vi "Horst-ZeitTest.vi"() -> ()   [LabVIEW 2017]
uses:
  <vilib>/rvi/interface/nirviMethod/nirviMethod.xnode
  E:/HAGAR-V_ECD/FPGA-Programm_ECD.vi
  <vilib>/FPGAPlugInAG/cRIO-9035/niLvFpga_WriteFifo_cRIO-9035.vi
  <vilib>/rvi/errors/niLvFpgaMergeErrorWithErrorCode.vi
  <vilib>/FPGAPlugInAG/cRIO-9035/niLvFpga_ReadFifo_cRIO-9035.vi
  <vilib>/rvi/interface/nirviReadWriteControl/nirviReadWriteControl.xnode
  <vilib>/rvi/interface/nirviCloseFPGA/nirviCloseFPGA.xnode
  <vilib>/regexp/Match Regular Expression.xnode
  GVECDs.vi
  FPGA Bitfiles/HAGAR-VECD_FPGATarget_FPGA-ProgrammECD_J-wKM9Jb3G8.lvbitx
  NiFpgaLv.dll
  <vilib>/Utility/error.llb/Error Cluster From Error Code.vi
  <vilib>/rvi/errors/niLvFpgaAdjustHostInterfaceError.vi
  <vilib>/FPGAPlugInAG/cRIO-9035/niLvFpga_Close_cRIO-9035.vi
panel:
  out "ECD2":string
  out "ECD1":string
  out "Array":errorcluster[](array[cluster])
  out "MW":dbl[](array[numeric])
  out "Fehler":bool[](array[boolean])
  in  "SP":dbl[](array[numeric]) format="%#_13g"
  in  "Stopp":bool
  out "stop":errorcluster caption="Fehler (Ausgang)"
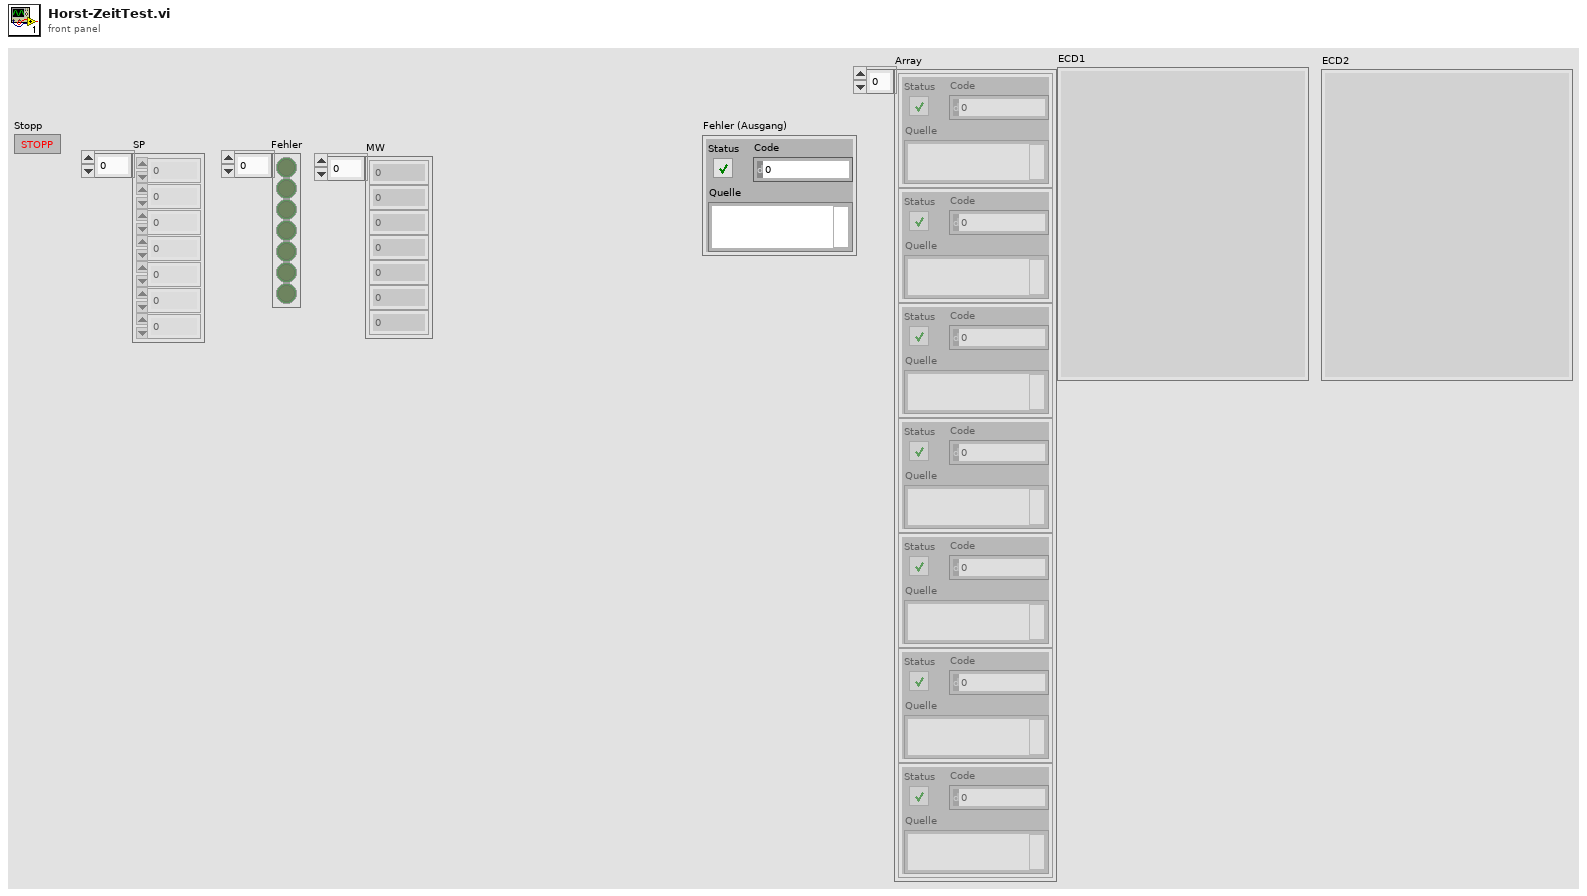
[diagram p1: front panel]
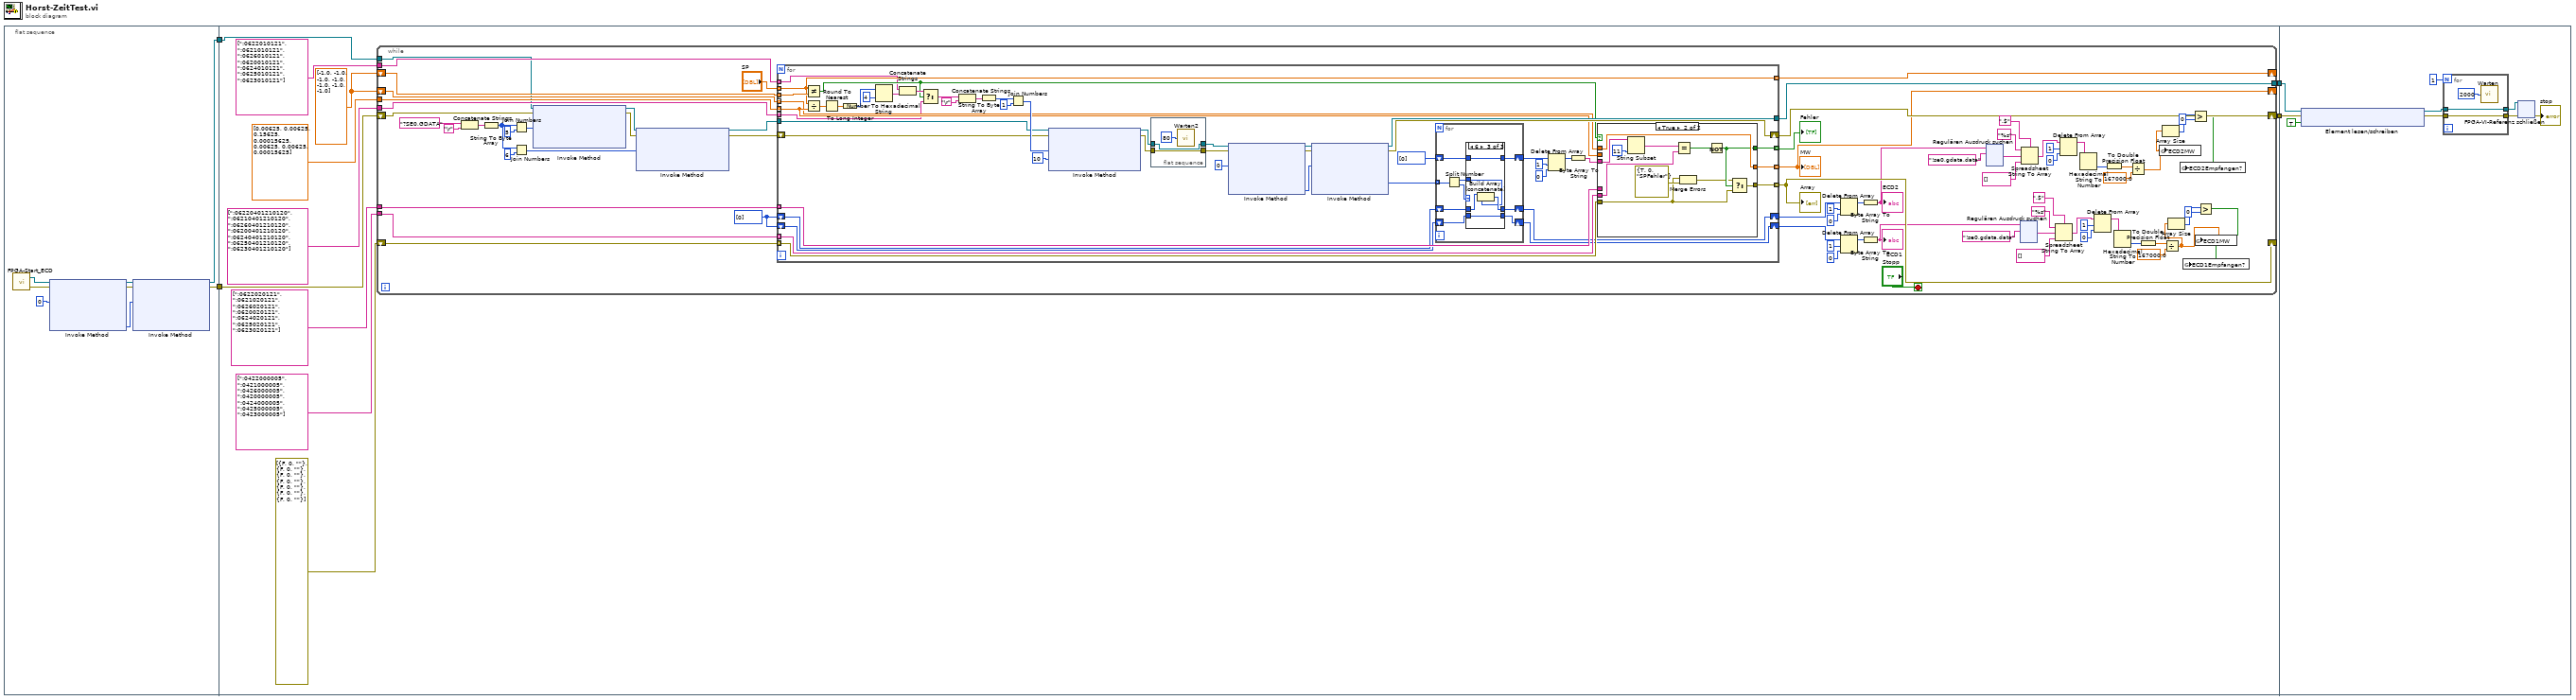
[diagram p0: block diagram]
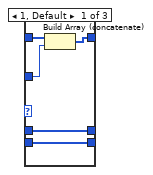
[diagram p2: hidden frame]
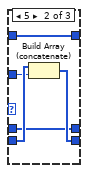
[diagram p3: hidden frame]
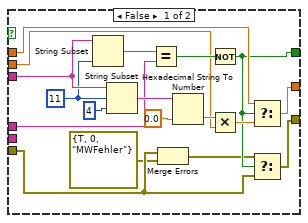
[diagram p4: hidden frame]
diagram:
  n1 = flat-sequence {
    tunnel: [w6] -> w4
    tunnel: [w5] -> w3
    tunnel: [w23] -> w2
    tunnel: [w22] -> w1
    tunnel: w4 -> [w21]
    tunnel: w3 -> [w20]
    tunnel: w2 -> [w425]
    tunnel: w1 -> [w424]
    frame #0 {
      n2 = call "FPGA-Start_ECD.vi"() -> ("error out"=w7:errorcluster, "FPGA-VI-Referenz (Ausgang)"=w8:refnum<k20>)  [unwired: 2 in]
      n3 = xnode "Invoke Method"("FPGA-VI-Referenz (Eingang)"=w8, "Fehler (Eingang)"=w7, "Anzahl der Elemente"=u32 0) -> ("FPGA-VI-Referenz (Ausgang)"=w12:refnum<k20>, "Fehler (Ausgang)"=w9:errorcluster, "Verbleibende Elemente"=w10:u32)  [unwired: 1 in, 1 out]
      n4 = xnode "Invoke Method"("FPGA-VI-Referenz (Eingang)"=w12, "Fehler (Eingang)"=w9, "Anzahl der Elemente"=w10) -> ("FPGA-VI-Referenz (Ausgang)"=w6:refnum<k20>, "Fehler (Ausgang)"=w5:errorcluster)  [unwired: 1 in, 2 out]
    }
    frame #1 {
      w19 = dbl[] [-1.0, -1.0, -1.0, -1.0, -1.0, -1.0, -1.0]
      n5 = while {
        shift-right: [w95] -> w22
        shift-left: w20 -> [w70]
        shift-right: [w92] -> _
        shift-left: w19 -> [w93]
        shift-right: [w89] -> _
        shift-left: w19 -> [w88]
        tunnel: string[] [":0622010121", ":0621010121", ":0626010121", ":0620010121", ":0624010121", ":0625010121", ":0623010121"] ("SPvorgebenMod2A") -> [w87]
        tunnel: string[] [":06220401210120", ":06210401210120", ":06260401210120", ":06200401210120", ":06240401210120", ":06250401210120", ":06230401210120"] ("MWabfragenMod2A") -> [w86]
        tunnel: dbl[] [0.00625, 0.00625, 0.15625, 0.00015625, 0.00625, 0.00625, 0.00015625] ("FaktorMod2A") -> [w85]
        tunnel: string[] [":0622020121", ":0621020121", ":0626020121", ":0620020121", ":0624020121", ":0625020121", ":0623020121"] ("MWAntwortMod2A") -> [w84]
        tunnel: string[] [":0422000005", ":0421000005", ":0426000005", ":0420000005", ":0424000005", ":0425000005", ":0423000005"] ("y") -> [w83]
        shift-right: [w82] -> _
        shift-left: errorcluster[] [{"status"=FALSE, "code"=0, "source"=""}, {"status"=FALSE, "code"=0, "source"=""}, {"status"=FALSE, "code"=0, "source"=""}, {"status"=FALSE, "code"=0, "source"=""}, {"status"=FALSE, "code"=0, "source"=""}, {"status"=FALSE, "code"=0, "source"=""}, {"status"=FALSE, "code"=0, "source"=""}] -> [w81]
        tunnel: w21 -> [w71]
        tunnel: [w96] -> w23
        stop <- "Stopp" stop-if-true
        w80 = u8[] [0]
        n6 = Concatenate Strings("?SE0,GDATA" ("Schreibpuffer"), "\r") -> (w59:string)
        n7 = String To Byte Array(string=w59) -> (unsigned byte array=w58:u8[])
        n8 = Join Numbers(hi=w58, lo=u8 5) -> ((hi.lo)=w63:u16[])
        n9 = Join Numbers(hi=w58, lo=u8 6) -> ((hi.lo)=w62:u16[])
        n10 = xnode "Invoke Method"("FPGA-VI-Referenz (Eingang)"=w71, "Fehler (Eingang)"=w70, "Daten"=w63) -> ("FPGA-VI-Referenz (Ausgang)"=w67:refnum<k20>, "Fehler (Ausgang)"=w65:errorcluster)  [unwired: 1 in, 1 out]
        n11 = xnode "Invoke Method"("FPGA-VI-Referenz (Eingang)"=w67, "Fehler (Eingang)"=w65, "Daten"=w62) -> ("FPGA-VI-Referenz (Ausgang)"=w66:refnum<k20>, "Fehler (Ausgang)"=w64:errorcluster)  [unwired: 1 in, 1 out]
        n12 = for {
          tunnel: w93 -> [w342] mode=indexing
          tunnel: [w338] -> w92 mode=indexing
          tunnel: [w339] -> w91 mode=indexing
          shift-right: [w362] -> w95
          shift-left: w64 -> [w354]
          tunnel: "SP" -> [w338] mode=indexing
          tunnel: w85 -> [w337] mode=indexing
          tunnel: [w336] -> w89 mode=indexing
          tunnel: w88 -> [w335] mode=indexing
          tunnel: w87 -> [w334] mode=indexing
          tunnel: w86 -> [w333] mode=indexing
          tunnel: w84 -> [w332] mode=indexing
          tunnel: w83 -> [w331] mode=indexing
          tunnel: [w330] -> w82 mode=indexing
          tunnel: w81 -> [w329] mode=indexing
          shift-right: [w319] -> w75
          shift-left: w80 -> [w322]
          shift-right: [w320] -> w74
          shift-left: w80 -> [w321]
          tunnel: w66 -> [w355]
          tunnel: [w365] -> w96
          n13 = Not Equal?(x=w338, y=w342) -> (x != y?=w340:bool)
          n14 = Divide(x=w338, y=w337) -> (x/y=w349:dbl)
          n15 = Round To Nearest(number=w349) -> (nearest integer value=w348:dbl)
          n16 = To Long Integer(number=w348) -> (32bit integer=w347:i32)
          n17 = Number To Hexadecimal String(1:i16 4 ("Breite (-)"), 2:w347) -> (0:w345:string)
          n18 = Concatenate Strings(w334, w345) -> (w344:string)
          n19 = Select(t=w344, s=w340, f=w333) -> (s? t:f=w343:string)
          n20 = Concatenate Strings(w343, "\r") -> (w361:string)
          n21 = String To Byte Array(string=w361) -> (unsigned byte array=w359:u8[])
          n22 = Join Numbers(hi=w359, lo=u8 1) -> ((hi.lo)=w360:u16[])
          n23 = xnode "Invoke Method"("FPGA-VI-Referenz (Eingang)"=w355, "Fehler (Eingang)"=w354, "Daten"=w360, "Timeout (ms)"=10) -> ("FPGA-VI-Referenz (Ausgang)"=w353:refnum<k20>, "Fehler (Ausgang)"=w351:errorcluster)  [unwired: 1 out]
          n24 = flat-sequence {
            tunnel: w353 -> [w423]
            tunnel: [w423] -> w352
            tunnel: w351 -> [w422]
            tunnel: [w422] -> w350
            frame #0 {
              n25 = call "Warten2"("Count(mSec)"=u32 80) -> ()  [unwired: 1 out]
            }
          }
          n26 = xnode "Invoke Method"("FPGA-VI-Referenz (Eingang)"=w352, "Fehler (Eingang)"=w350, "Anzahl der Elemente"=u32 0) -> ("FPGA-VI-Referenz (Ausgang)"=w364:refnum<k20>, "Fehler (Ausgang)"=w363:errorcluster, "Verbleibende Elemente"=w366:u32)  [unwired: 1 in, 1 out]
          n27 = xnode "Invoke Method"("FPGA-VI-Referenz (Eingang)"=w364, "Fehler (Eingang)"=w363, "Anzahl der Elemente"=w366) -> ("FPGA-VI-Referenz (Ausgang)"=w365:refnum<k20>, "Fehler (Ausgang)"=w362:errorcluster, "Daten"=w328:u16[])  [unwired: 1 in, 1 out]
          n28 = for {
            tunnel: w328 -> [w376] mode=indexing
            shift-right: [w370] -> w326
            shift-left: u8[] [0] -> [w371]
            shift-right: [w369] -> w319
            shift-left: w322 -> [w372]
            shift-right: [w368] -> w320
            shift-left: w321 -> [w373]
            n29 = Split Number(x=w376) -> (hi(x)=w374:u8, lo(x)=w375:u8)
            n30 = case shown="6" w375 {
              tunnel: w374 -> [w381 w384 w387]
              tunnel: w373 -> [w377 w382 w390]
              tunnel: w372 -> [w378 w385 w389]
              tunnel: w371 -> [w380 w386 w391]
              tunnel: [w379 w386 w391] -> w370
              tunnel: [w378 w383 w389] -> w369
              tunnel: [w377 w382 w388] -> w368
              frame 1, Default {
                n31 = Build Array (concatenate)(w380, w381) -> (w379:u8[])
              }
              frame 5 {
                n32 = Build Array (concatenate)(w385, w384) -> (w383:u8[])
              }
              frame 6 {
                n33 = Build Array (concatenate)(w390, w387) -> (w388:u8[])
              }
            }
          }
          n34 = Delete From Array(array=w326, length=1 ("Länge"), index=0 ("Index")) -> (array with subset deleted=w323:u8[])  [unwired: 1 out]
          n35 = Byte Array To String(unsigned byte array=w323) -> (string=w341:string)
          n36 = case shown="True" w340 {
            tunnel: w341 -> [w407 w420]
            tunnel: [w396 w414] -> w339
            tunnel: w337 -> [w401 _]
            tunnel: [w398 w416] -> w336
            tunnel: w335 -> [w399 w416]
            tunnel: w332 -> [w397 _]
            tunnel: w331 -> [_ w415]
            tunnel: [w395 w413] -> w330
            tunnel: w329 -> [w394 w410]
            frame False {
              w406 = 11 ("Länge (Rest)")
              n37 = String Subset(string=w407, length (rest)=w406) -> (substring=w409:string)  [unwired: 1 in]
              n38 = String Subset(string=w407, offset (0)=w406, length (rest)=4 ("Länge (Rest)")) -> (substring=w404:string)
              n39 = Equal?(x=w409, y=w397) -> (x = y?=w408:bool)
              n40 = Merge Errors(w394, errorcluster {"status"=TRUE, "code"=0, "source"="MWFehler"} ("Fehlerkonstante")) -> (w393:errorcluster)
              n41 = Hexadecimal String To Number(string=w404, default (0uL)=0.0 ("Standard (0 U32)")) -> (number=w402:dbl)  [unwired: 1 in, 1 out]
              n42 = Not(x=w408) -> (.not. x?=w396:bool)
              n43 = Multiply(x=w402, y=w401) -> (x*y=w400:dbl)
              n44 = Select(t=w399, s=w396, f=w400) -> (s? t:f=w398:dbl)
              n45 = Select(t=w393, s=w396, f=w394) -> (s? t:f=w395:errorcluster)
            }
            frame True {
              n46 = String Subset(string=w420, length (rest)=11 ("Länge (Rest)")) -> (substring=w419:string)  [unwired: 1 in]
              n47 = Equal?(x=w419, y=w415) -> (x = y?=w417:bool)
              n48 = Merge Errors(w410, errorcluster {"status"=TRUE, "code"=0, "source"="SPFehler"} ("Fehler (Eingang)")) -> (w411:errorcluster)
              n49 = Not(x=w417) -> (.not. x?=w414:bool)
              n50 = Select(t=w411, s=w414, f=w410) -> (s? t:f=w413:errorcluster)
            }
          }
        }
        "Fehler" <- w91
        "MW" <- w89
        "Array" <- w82
        n51 = Delete From Array(array=w74, length=1 ("Länge"), index=0 ("Index")) -> (array with subset deleted=w72:u8[])  [unwired: 1 out]
        n52 = Delete From Array(array=w75, length=1 ("Länge"), index=0 ("Index")) -> (array with subset deleted=w73:u8[])  [unwired: 1 out]
        n53 = Byte Array To String(unsigned byte array=w72) -> (string=w32:string)
        "ECD2" <- w32
        n54 = Byte Array To String(unsigned byte array=w73) -> (string=w50:string)
        "ECD1" <- w50
        n55 = xnode "Regulären Ausdruck suchen"("Eingangs-String"=w32, "Regulärer Ausdruck"="!se0,gdata,data") -> ("Nach Übereinstimmung"=w38:string)  [unwired: 4 in, 4 out]
        n56 = xnode "Regulären Ausdruck suchen"("Eingangs-String"=w50, "Regulärer Ausdruck"="!se0,gdata,data") -> ("Nach Übereinstimmung"=w51:string)  [unwired: 4 in, 4 out]
        n57 = Spreadsheet String To Array(delimiter (Tab)=",$" ("Trennzeichen (Tabulator)"), format string="%s" ("Format-String"), spreadsheet string=w38, array type (2D Dbl)=string[] []) -> (array=w35:string[])
        n58 = Spreadsheet String To Array(delimiter (Tab)=",$" ("Trennzeichen (Tabulator)"), format string="%s" ("Format-String"), spreadsheet string=w51, array type (2D Dbl)=string[] []) -> (array=w47:string[])
        n59 = Delete From Array(array=w35, length=1 ("Länge"), index=0 ("Index")) -> (array with subset deleted=w33:string[])  [unwired: 1 out]
        n60 = Hexadecimal String To Number(string=w33) -> (number=w41:u32[])  [unwired: 2 in, 1 out]
        n61 = Delete From Array(array=w47, length=1 ("Länge"), index=0 ("Index")) -> (array with subset deleted=w45:string[])  [unwired: 1 out]
        n62 = To Double Precision Float(number=w41) -> (double precision float=w40:dbl[])
        n63 = Hexadecimal String To Number(string=w45) -> (number=w54:u32[])  [unwired: 2 in, 1 out]
        n64 = Divide(x=w40, y=167000.0) -> (x/y=w25:dbl[])
        n65 = To Double Precision Float(number=w54) -> (double precision float=w53:dbl[])
        n66 = global write "GVECDs.vi" "ECD2MW"(w25) -> ()
        n67 = Array Size(array=w25) -> (size(s)=w27:i32)
        n68 = Divide(x=w53, y=167000.0) -> (x/y=w31:dbl[])
        n69 = Array Size(array=w31) -> (size(s)=w30:i32)
        n70 = Greater?(x=w27, y=0) -> (0:w24:bool)
        n71 = global write "GVECDs.vi" "ECD2Empfangen?"(w24) -> ()
        n72 = global write "GVECDs.vi" "ECD1MW"(w31) -> ()
        n73 = Greater?(x=w30, y=0) -> (0:w28:bool)
        n74 = global write "GVECDs.vi" "ECD1Empfangen?"(w28) -> ()
      }
    }
    frame #2 {
      n75 = xnode "Element lesen/schreiben"("FPGA-VI-Referenz (Eingang)"=w425, "Fehler (Eingang)"=w424, "global stop"=TRUE) -> ("FPGA-VI-Referenz (Ausgang)"=w428:refnum<k20>, "Fehler (Ausgang)"=w429:errorcluster)
      n76 = for {
        N: 1 -> [_]
        tunnel: w428 -> [w434]
        tunnel: w429 -> [w433]
        tunnel: [w434] -> w430
        tunnel: [w433] -> w431
        n77 = call "Warten"("Count(mSec)"=u32 2000) -> ()  [unwired: 1 out]
      }
      n78 = xnode "FPGA-VI-Referenz schließen"("FPGA-VI-Referenz (Eingang)"=w430, "Fehler (Eingang)"=w431) -> ("Fehler (Ausgang)"=→"stop":errorcluster)
    }
  }
